vi "stage_getposition.vi"(8 "error in (no error)":errorcluster, 11 "Stage reference in":T2) -> (0 "error out":errorcluster, 2 "position":T1, 3 "Stage reference out":T2)   [LabVIEW 2018]
uses:
  stage_reference_type.ctl
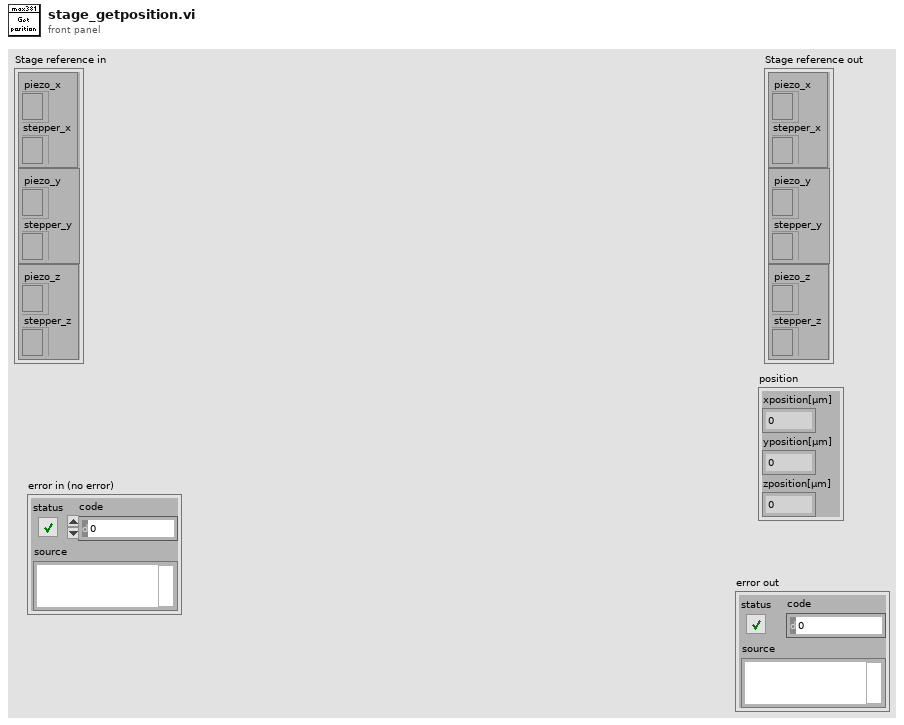
[diagram p1: front panel]
types:
  T1 = cluster{"xposition[µm]":sgl, "yposition[µm]":sgl, "zposition[µm]":sgl}
  T2 = typedef "stage_reference_type.ctl" = cluster{cluster{"piezo_x":refnum<k7>, "stepper_x":refnum<k7>}, cluster{"piezo_y":refnum<k7>, "stepper_y":refnum<k7>}, cluster{"piezo_z":refnum<k7>, "stepper_z":refnum<k7>}}
  T3 = cluster{"piezo_x":refnum<k7>, "stepper_x":refnum<k7>}
  T4 = cluster{"piezo_y":refnum<k7>, "stepper_y":refnum<k7>}
  T5 = cluster{"piezo_z":refnum<k7>, "stepper_z":refnum<k7>}
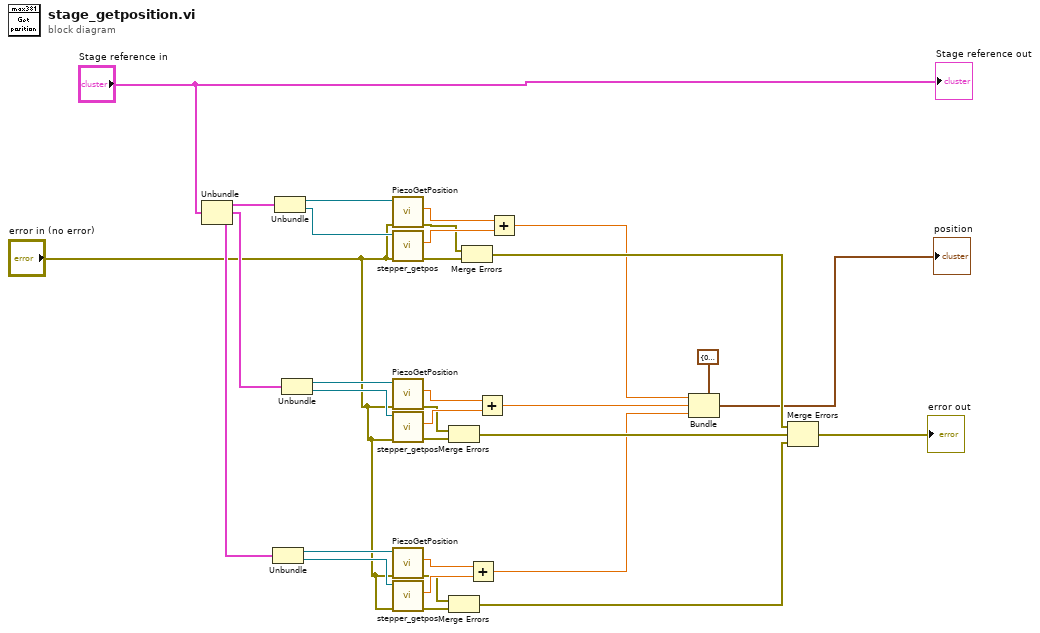
[diagram p0: block diagram]
diagram:
  n1 = Unbundle("Stage reference in") -> (w31:T3, w30:T4, w29:T5)
  n2 = Unbundle(w29) -> ("piezo_z"=w25:refnum<k7>, "stepper_z"=w12:refnum<k7>)
  n3 = Unbundle(w31) -> ("piezo_x"=w28:refnum<k7>, "stepper_x"=w27:refnum<k7>)
  n4 = Unbundle(w30) -> ("piezo_y"=w26:refnum<k7>, "stepper_y"=w11:refnum<k7>)
  n5 = call <userlib>:"PiezoGetPosition.vi"("error in (no error)"="error in (no error)", "reference"=w28) -> ("error out"=w18:errorcluster, "Position"=w24:sgl)  [unwired: 3 in, 1 out]
  n6 = call <userlib>:"stepper_getpos.vi"("error in (no error)"="error in (no error)", "reference"=w27) -> ("error out"=w17:errorcluster, "pfPosition[µm]"=w23:sgl)  [unwired: 7 in, 1 out]
  n7 = call <userlib>:"PiezoGetPosition.vi"("error in (no error)"="error in (no error)", "reference"=w26) -> ("error out"=w16:errorcluster, "Position"=w22:sgl)  [unwired: 3 in, 1 out]
  n8 = call <userlib>:"stepper_getpos.vi"("error in (no error)"="error in (no error)", "reference"=w11) -> ("error out"=w15:errorcluster, "pfPosition[µm]"=w21:sgl)  [unwired: 7 in, 1 out]
  n9 = call <userlib>:"PiezoGetPosition.vi"("error in (no error)"="error in (no error)", "reference"=w25) -> ("error out"=w14:errorcluster, "Position"=w20:sgl)  [unwired: 3 in, 1 out]
  n10 = call <userlib>:"stepper_getpos.vi"("error in (no error)"="error in (no error)", "reference"=w12) -> ("error out"=w13:errorcluster, "pfPosition[µm]"=w19:sgl)  [unwired: 7 in, 1 out]
  n11 = Merge Errors(w16, w15) -> (w9:errorcluster)
  n12 = Merge Errors(w14, w13) -> (w8:errorcluster)
  n13 = Merge Errors(w18, w17) -> (w10:errorcluster)
  n14 = Add(x=w20, y=w19) -> (x+y=w3:sgl)
  n15 = Add(x=w22, y=w21) -> (x+y=w4:sgl)
  n16 = Add(x=w24, y=w23) -> (x+y=w2:sgl)
  n17 = Bundle(cluster=T1 {"xposition[µm]"=0.0, "yposition[µm]"=0.0, "zposition[µm]"=0.0} ("output cluster"), "xposition[µm]"=w2, "yposition[µm]"=w4, "zposition[µm]"=w3) -> (→"position":T1)
  n18 = Merge Errors(w10, w9, w8) -> (→"error out":errorcluster)
  "Stage reference out" <- "Stage reference in"
